vi "SBPB.vi"(0 "Rate(ms)":u16=1 max=9999 format="%#.0f", 3 "coupling distance(x0.1um)":u32, 4 "y-dist":i32, 5 "x-before(x0.1um)":u32, 6 "Motor GPIB":u8=6, 7 "Current (mA)":dbl, 8 "speed":u16, 9 "x-dist":i32, 10 "Laser GPIB":u8=10 max=100) -> ()   [LabVIEW 2010]
uses:
  <vilib>/express/express arith-compare/Formula/XNode/ExpressFormulaBlockNode.xnode
panel:
  out "dummy":string
  # "7) SBENDP<space>[x-disp];[Speed];[Current]<space>[x_before];[coupling_distance]<space>[y-disp];[rate]"
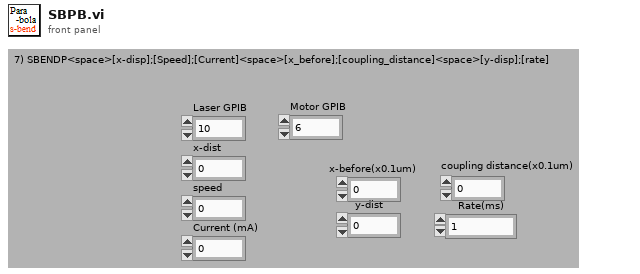
[diagram p1: front panel]
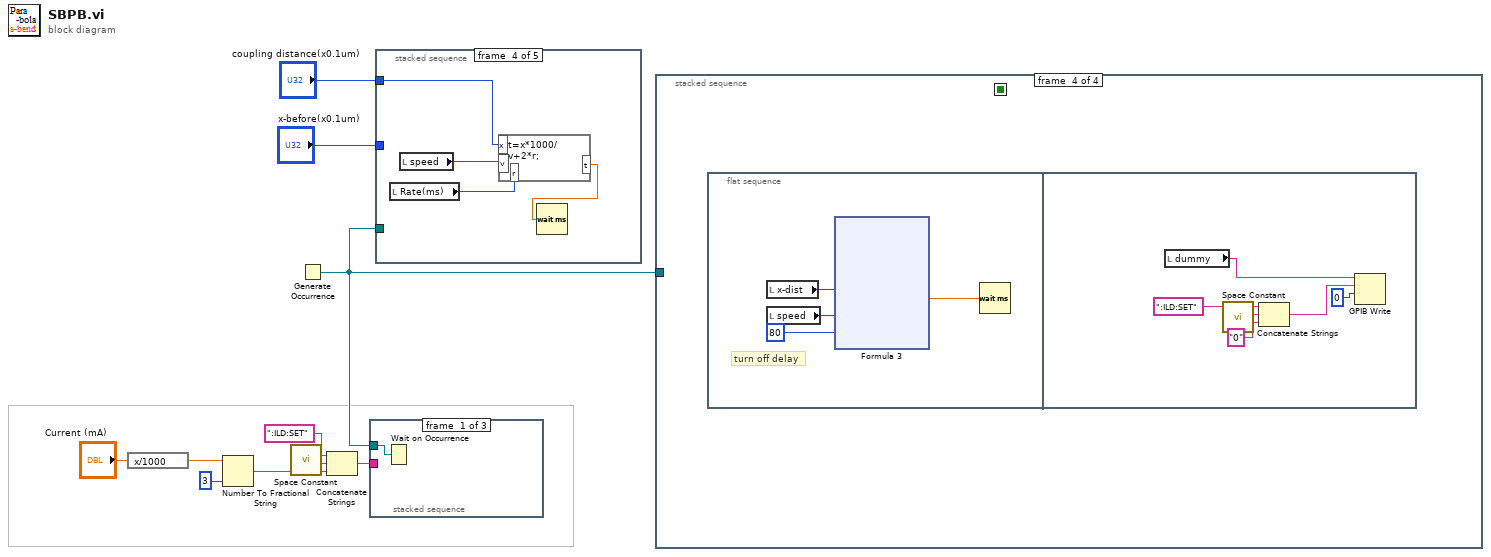
[diagram p0: block diagram]
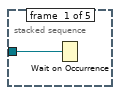
[diagram p2: hidden frame]
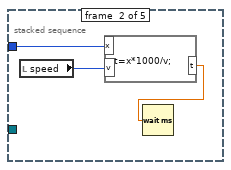
[diagram p3: hidden frame]
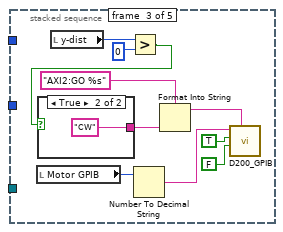
[diagram p4: hidden frame]
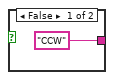
[diagram p5: hidden frame]
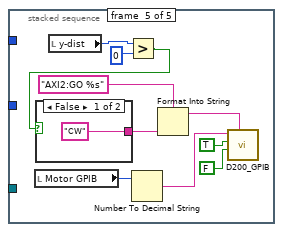
[diagram p6: hidden frame]
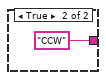
[diagram p7: hidden frame]
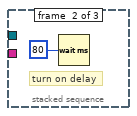
[diagram p8: hidden frame]
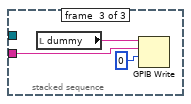
[diagram p9: hidden frame]
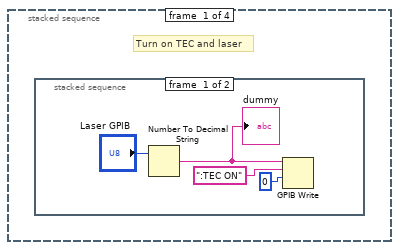
[diagram p10: hidden frame]
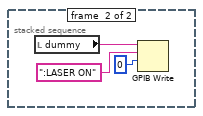
[diagram p11: hidden frame]
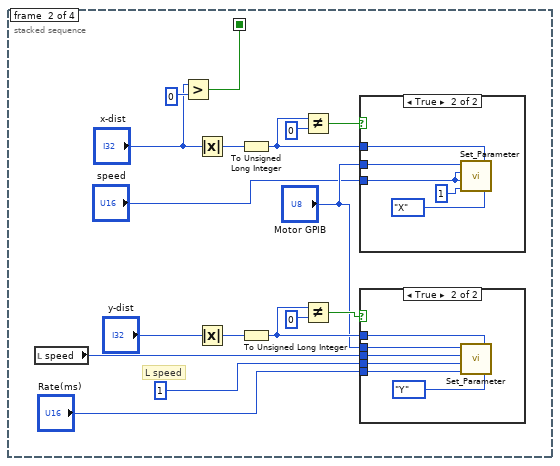
[diagram p12: hidden frame]
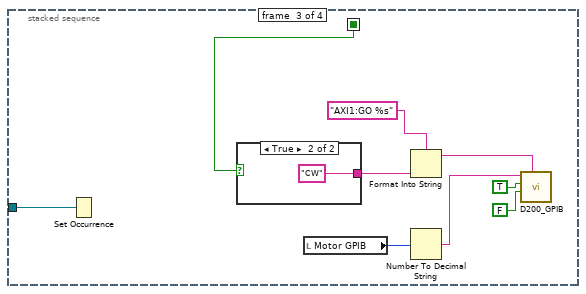
[diagram p15: hidden frame]
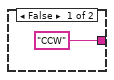
[diagram p16: hidden frame]
diagram:
  n1 = expression code="x/1000"("Current (mA)") -> (w4:dbl)
  n2 = Number To Fractional String(number=w4, precision (6)=i16 3) -> (F-format string=w7:string)  [unwired: 2 in]
  n3 = call <vilib>:"Space Constant.vi"() -> ("String"=w9:string)
  n4 = Generate Occurrence() -> (w3:refnum<k4>)
  n5 = Concatenate Strings(":ILD:SET", w9, w7) -> (w10:string)
  n6 = stacked-sequence {
    tunnel: w10 -> [_ _ w13]
    tunnel: w3 -> [w11 _ _]
    frame #0 {
      n7 = Wait on Occurrence(2:w11) -> ()  [unwired: 2 in, 1 out]
    }
    frame #1 {
      # "turn on delay"
      n8 = Wait (ms)(milliseconds to wait=u16 80 ("X4")) -> ()  [unwired: 1 out]
    }
    frame #2 {
      n9 = local read "dummy"() -> (w15:string)
      n10 = GPIB Write(0:w15, 1:w13, 2:i16 0 ("mode (0)")) -> ()  [unwired: 2 in, 2 out]
    }
  }
  n11 = stacked-sequence {
    tunnel: w3 -> [w16 _ _ _ _]
    tunnel: "x-before(x0.1um)" -> [_ w18 _ _ _]
    tunnel: "coupling distance(x0.1um)" -> [_ _ _ w33 _]
    frame #0 {
      n12 = Wait on Occurrence(2:w16) -> ()  [unwired: 2 in, 1 out]
    }
    frame #1 {
      n13 = local read "speed"() -> (w17:u16)
      n14 = formula code="t=x*1000/v;"("x"=w18, "v"=w17) -> ("t"=w19:dbl)
      n15 = Wait (ms)(milliseconds to wait=w19) -> ()  [unwired: 1 out]
    }
    frame #2 {
      n16 = local read "Motor GPIB"() -> (w29:u8)
      n17 = local read "y-dist"() -> (w20:i32)
      n18 = Greater?(x=w20, y=0) -> (0:w21:bool)
      n19 = case shown="True" w21 {
        tunnel: ["CCW" "CW"] -> w27
        frame False {
        }
        frame True {
        }
      }
      n20 = Number To Decimal String(number=w29) -> (decimal integer string=w23:string)  [unwired: 1 in]
      n21 = Format Into String(format string="AXI2:GO %s", w27) -> (resulting string=w24:string)  [unwired: 2 in, 1 out]
      n22 = call "D200_GPIB.vi"("GPIB\nAddress"=w23, "Write"=TRUE, "Read"=FALSE, "Characters to Write"=w24) -> ()  [unwired: 1 in, 3 out]
    }
    frame #3 {
      n23 = local read "Rate(ms)"() -> (w32:u16)
      n24 = local read "speed"() -> (w34:u16)
      n25 = formula code="t=x*1000/v+2*r;"("x"=w33, "v"=w34, "r"=w32) -> ("t"=w35:dbl)
      n26 = Wait (ms)(milliseconds to wait=w35) -> ()  [unwired: 1 out]
    }
    frame #4 {
      n27 = local read "Motor GPIB"() -> (w45:u8)
      n28 = local read "y-dist"() -> (w36:i32)
      n29 = Greater?(x=w36, y=0) -> (0:w37:bool)
      n30 = case shown="False" w37 {
        tunnel: ["CW" "CCW"] -> w43
        frame False {
        }
        frame True {
        }
      }
      n31 = Number To Decimal String(number=w45) -> (decimal integer string=w39:string)  [unwired: 1 in]
      n32 = Format Into String(format string="AXI2:GO %s", w43) -> (resulting string=w40:string)  [unwired: 2 in, 1 out]
      n33 = call "D200_GPIB.vi"("GPIB\nAddress"=w39, "Write"=TRUE, "Read"=FALSE, "Characters to Write"=w40) -> ()  [unwired: 1 in, 3 out]
    }
  }
  n34 = stacked-sequence {
    seq-local: [_ w56 _ _] -> [_ _ w83 _]
    tunnel: w3 -> [_ _ w91 _]
    frame #0 {
      # "Turn on TEC and laser"
      n35 = stacked-sequence {
        frame #0 {
          n36 = Number To Decimal String(number="Laser GPIB") -> (decimal integer string=w48:string)  [unwired: 1 in]
          "dummy" <- w48
          n37 = GPIB Write(0:w48, 1:":TEC ON" ("data"), 2:i16 0 ("mode (0)")) -> ()  [unwired: 2 in, 2 out]
        }
        frame #1 {
          n38 = local read "dummy"() -> (w53:string)
          n39 = GPIB Write(0:w53, 1:":LASER ON" ("data"), 2:i16 0 ("mode (0)")) -> ()  [unwired: 2 in, 2 out]
        }
      }
    }
    frame #1 {
      # "L speed"
      n40 = local read "speed"() -> (w55:u16)
      n41 = Greater?(x="x-dist", y=0) -> (0:w56:bool)
      n42 = Absolute Value(x="x-dist") -> (abs(x)=w71:i32)
      n43 = Absolute Value(x="y-dist") -> (abs(x)=w64:i32)
      n44 = To Unsigned Long Integer(number=w71) -> (unsigned 32bit integer=w70:u32)
      n45 = To Unsigned Long Integer(number=w64) -> (unsigned 32bit integer=w65:u32)
      n46 = Not Equal?(x=w70, y=u32 0) -> (x != y?=w68:bool)
      n47 = Not Equal?(x=w65, y=u32 0) -> (x != y?=w67:bool)
      n48 = case shown="True" w68 {
        tunnel: "Motor GPIB" -> [_ w82]
        tunnel: w70 -> [_ w79]
        tunnel: "speed" -> [_ w78]
        frame False {
        }
        frame True {
          n49 = call "Set_Parameter.vi"("Axis"=enum16{"X", "Y", "Z", "U", "V", "W"}."X", "Distance"=w79, "Rate"=u16 1, "L Speed"=w78, "F Speed"=w78, "GPIB_Addr"=w82) -> ()
        }
      }
      n50 = case shown="True" w67 {
        tunnel: "Motor GPIB" -> [_ w77]
        tunnel: w65 -> [_ w75]
        tunnel: w55 -> [_ w74]
        tunnel: u16 1 ("L Speed") -> [_ w73]
        tunnel: "Rate(ms)" -> [_ w72]
        frame False {
        }
        frame True {
          n51 = call "Set_Parameter.vi"("Axis"=enum16{"X", "Y", "Z", "U", "V", "W"}."Y", "Distance"=w75, "Rate"=w72, "L Speed"=w73, "F Speed"=w74, "GPIB_Addr"=w77) -> ()
        }
      }
    }
    frame #2 {
      n52 = Set Occurrence(w91) -> ()
      n53 = case shown="True" w83 {
        tunnel: ["CCW" "CW"] -> w86
        frame False {
        }
        frame True {
        }
      }
      n54 = local read "Motor GPIB"() -> (w84:u8)
      n55 = Format Into String(format string="AXI1:GO %s", w86) -> (resulting string=w89:string)  [unwired: 2 in, 1 out]
      n56 = Number To Decimal String(number=w84) -> (decimal integer string=w90:string)  [unwired: 1 in]
      n57 = call "D200_GPIB.vi"("GPIB\nAddress"=w90, "Write"=TRUE, "Read"=FALSE, "Characters to Write"=w89) -> ()  [unwired: 1 in, 3 out]
    }
    frame #3 {
      n58 = flat-sequence {
        frame #0 {
          # "turn off delay"
          n59 = local read "x-dist"() -> (w96:i32)
          n60 = local read "speed"() -> (w95:u16)
          n61 = xnode "Formula 3"("x_dist"=w96, "speed"=w95, "delay"=u16 80 ("X4")) -> ("Result"=w97:dbl)  [unwired: 1 in, 1 out]
          n62 = Wait (ms)(milliseconds to wait=w97) -> ()  [unwired: 1 out]
        }
        frame #1 {
          n63 = local read "dummy"() -> (w110:string)
          n64 = call <vilib>:"Space Constant.vi"() -> ("String"=w113:string)
          n65 = Concatenate Strings(":ILD:SET", w113, "0" ("string")) -> (w112:string)
          n66 = GPIB Write(0:w110, 1:w112, 2:i16 0 ("mode (0)")) -> ()  [unwired: 2 in, 2 out]
        }
      }
    }
  }
